vi "PH_PP_CurrentMeas.destructor.vi"(0 "i ref in":refnum<vi>, 5 "error in(no error)":errorcluster) -> (19 "error out":errorcluster)   [LabVIEW 2014, in "PH_PP_CurrentMeas.lvlib"]
doc: "This is the destructor of a class.\n\nLicense Agreement for this software:\n\nCopyright (C)\nGesellschaft für Schwerionenforschung, GSI\nPlanckstr. 1\n64291 Darmstadt\nGermany\n\nContact: D.Beck@gsi.de \n\nThis program is free software; you can redistribute it and/or modify it under the terms of the \nGNU General Public License as published by the Free Software Foundation; either version 2 of \nthe license, or (at your option) any later version.\n\nThis program is distributed in the hope that it will be useful, but WITHOUT ANY WARRANTY; \nwithout even the implied warranty of MERCHANTABILITY or FITNESS FOR A PARTICULAR PURPOSE. See the GNU General License for more details (http://www.gnu.org).\n\nGesellschaft für Schwerionenforschung, GSI\nPlanckstr. 1, 64291 Darmstadt, Germany\nFor all questions and ideas contact: M.Richter@gsi.de, H.Brand@gsi.de or D.Beck@gsi.de.\nLast update: 16-JUN-2004"
uses:
  PH_PP_CurrentMeas.lvlib
  PH_PSDBWriter/PH_PSDBWriter.lvlib
  PH_StatusHandler/PH_StatusHandler.lvlib
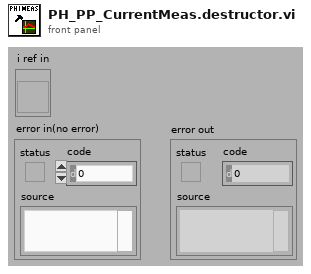
[diagram p1: front panel]
types:
  T1 = enum16{"SetAttribute", "GetAttribute", "CreateAttribute", "DestroyAttribute", "DestroyAllAtributes"}
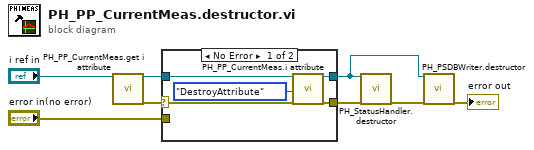
[diagram p0: block diagram]
diagram:
  n1 = call "PH_PP_CurrentMeas.get i attribute.vi"("i ref in"="i ref in") -> ("i ref out"=w6:refnum<vi>, "error out"=w2:errorcluster)  [unwired: 16 in, 1 out]
  n2 = case shown="No Error" w2 {
    selector: w2 -> [w9 _]
    tunnel: [w12 w15] -> w7
    tunnel: w6 -> [w11 w14]
    tunnel: [w10 w14] -> w3
    tunnel: "error in(no error)" -> [_ w15]
    frame No Error {
      n3 = call "PH_PP_CurrentMeas.i attribute.vi"("VI Refnum"=w11, "Action"=T1."DestroyAttribute", "error in (no error)"=w9) -> ("VI Refnum out"=w10:refnum<vi>, "error out"=w12:errorcluster)  [unwired: 14 in, 1 out]
    }
    frame Error {
    }
  }
  n4 = call "PH_StatusHandler.destructor.vi"("i ref in"=w3, "error in(no error)"=w7) -> ("error out"=w4:errorcluster)  [unwired: 17 in]
  n5 = call "PH_PSDBWriter.destructor.vi"("i ref in"=w3, "error in(no error)"=w4) -> ("error out"=→"error out":errorcluster)  [unwired: 17 in]
